vi "oa_Perform RMS Averaging (1 Channel).vi"(6 "averaging state info in":T1 {"averages completed" format="%.2f"; "power spectrum" min=0.0 max=127.0 format="%.2f"; "complex FFT" format="%.2f"}, 7 "processing control in":T2(ring), 8 "error in (no error)":errorcluster, 9 "averaging parameters":T3={"averaging mode"=enum."No averaging", "weighting mode"=enum."Exponential", "number of averages"=10, "linear mode"=enum."One shot"} {"number of averages" min=1 step=1}, 11 "Y":dbl[][](array[numeric]) format="%.2f") -> (0 "error out":errorcluster, 1 "averages completed":dbl, 2 "averaging done":bool, 3 "Y out":dbl[](array[numeric]) format="%.2f", 4 "averaging state info out":T1 {"averages completed" format="%.2f"; "power spectrum" min=0.0 max=127.0 format="%.2f"; "complex FFT" format="%.2f"})   [LabVIEW 2017, in "SoundVib_Resampling.lvlib"]
uses:
  <vilib>/addons/Sound and Vibration/Order Analysis/Resample Order Tracking/SoundVib_Resampling.lvlib
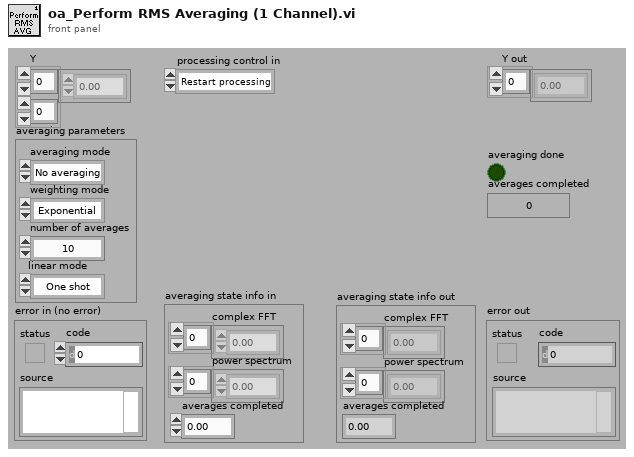
[diagram p1: front panel]
types:
  T1 = cluster{"complex FFT":cdb[], "power spectrum":dbl[], "averages completed":dbl}
  T2 = enum16{"Restart processing", "Continue processing", "Skip processing"}
  T3 = cluster{"averaging mode":enum16{"No averaging", "Vector averaging", "RMS averaging", "Peak hold"}, "weighting mode":enum16{"Linear", "Exponential"}, "number of averages":u32, "linear mode":enum16{"One shot", "Auto restart"}}
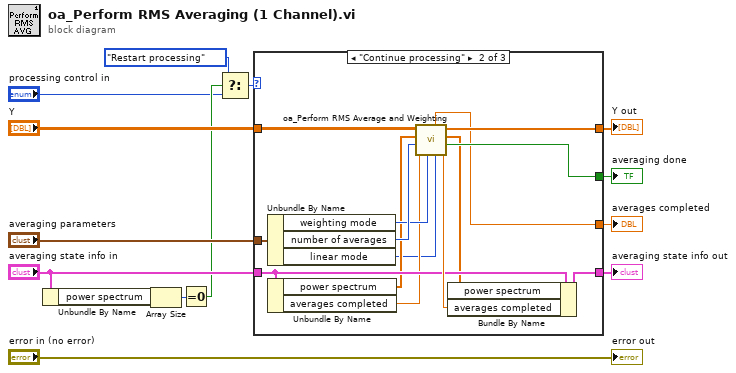
[diagram p0: block diagram]
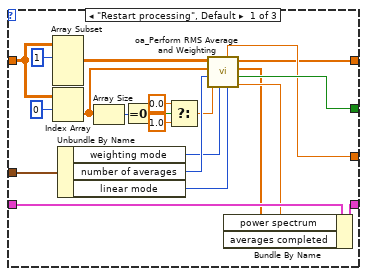
[diagram p2: hidden frame]
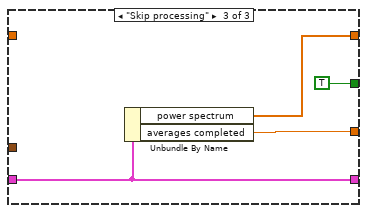
[diagram p3: hidden frame]
diagram:
  n1 = Unbundle By Name("averaging state info in") -> ("power spectrum"=w7:dbl[])
  n2 = Array Size(array=w7) -> (size(s)=w6:i32)
  n3 = Equal To 0?(x=w6) -> (x = 0?=w4:bool)
  n4 = Select(t=T2."Restart processing", s=w4, f="processing control in") -> (s? t:f=w3:T2)
  n5 = case shown="\"Continue processing\"" w3 {
    tunnel: "averaging parameters" -> [w33 w41 _]
    tunnel: "Y" -> [w23 w47 _]
    tunnel: "averaging state info in" -> [w35 w43 w52]
    tunnel: [w34 w44 w52] -> w12
    tunnel: [w17 w36 w51] -> w11
    tunnel: [w31 w46 TRUE] -> w10
    tunnel: [w16 w38 w50] -> w8
    frame "Restart processing", Default {
      n6 = Array Subset(array=w23, index (row)=1 ("index")) -> (w22:dbl[][])  [unwired: 3 in]
      n7 = Index Array(array=w23, index (row)=0) -> (element=w21:dbl[])  [unwired: 1 in]
      n8 = Unbundle By Name(w33) -> ("weighting mode"=w29:enum16{"Linear", "Exponential"}, "number of averages"=w32:u32, "linear mode"=w18:enum16{"One shot", "Auto restart"})
      n9 = Array Size(array=w21) -> (size(s)=w26:i32)
      n10 = Equal To 0?(x=w26) -> (x = 0?=w19:bool)
      n11 = Select(t=0.0, s=w19, f=1.0) -> (s? t:f=w20:dbl)
      n12 = call <vilib>:"oa_Perform RMS Average and Weighting.vi"("linear mode"=w18, "weighting mode"=w29, "averages completed"=w20, "number of averages"=w32, "previous array"=w21, "Y"=w22) -> ("averages completed for buffer"=w30:dbl, "average done?"=w31:bool, "power spectrum for buffer"=w15:dbl[], "power spectrum for output"=w16:dbl[], "averages completed for output"=w17:dbl)  [unwired: 1 in]
      n13 = Bundle By Name(cluster=w35, "power spectrum"=w15, "averages completed"=w30) -> (w34:T1)
    }
    frame "Continue processing" {
      n14 = Unbundle By Name(w41) -> ("weighting mode"=w48:enum16{"Linear", "Exponential"}, "number of averages"=w49:u32, "linear mode"=w39:enum16{"One shot", "Auto restart"})
      n15 = Unbundle By Name(w43) -> ("power spectrum"=w42:dbl[], "averages completed"=w40:dbl)
      n16 = call <vilib>:"oa_Perform RMS Average and Weighting.vi"("linear mode"=w39, "weighting mode"=w48, "averages completed"=w40, "number of averages"=w49, "previous array"=w42, "Y"=w47) -> ("averages completed for buffer"=w45:dbl, "average done?"=w46:bool, "power spectrum for buffer"=w37:dbl[], "power spectrum for output"=w38:dbl[], "averages completed for output"=w36:dbl)  [unwired: 1 in]
      n17 = Bundle By Name(cluster=w43, "power spectrum"=w37, "averages completed"=w45) -> (w44:T1)
    }
    frame "Skip processing" {
      n18 = Unbundle By Name(w52) -> ("power spectrum"=w50:dbl[], "averages completed"=w51:dbl)
    }
  }
  "averaging done" <- w10
  "averages completed" <- w11
  "Y out" <- w8
  "averaging state info out" <- w12
  "error out" <- "error in (no error)"
